vi "Get Time.vi"(9 "Next State in":T1, 10 "Current State":T1, 11 "State Start Time in":u32) -> (1 "Next State out":T1, 2 "Reset":bool, 3 "State Start Time out":u32)   [LabVIEW 2013]
uses:
  Auto Two Ball States.ctl
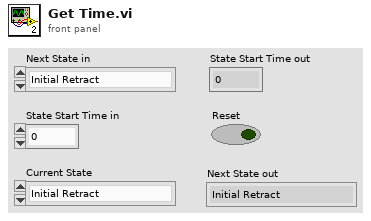
[diagram p1: front panel]
types:
  T1 = typedef "Auto Two Ball States.ctl" = enum16{"Initial Retract", "Initial Retract Wait", "First Shot: Wait for ball", "First Shot: Shoot", "Second Shot: Wait for Arm", "Grab Second Ball", "Grab Second Ball Wait", "Second Shot: Wait for ball", "Second Shot: Shoot", "Drive Forward", "Finish"}
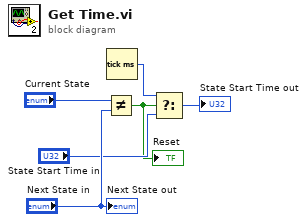
[diagram p0: block diagram]
diagram:
  n1 = Not Equal?(x="Current State", y="Next State in") -> (x != y?=w3:bool)
  "Reset" <- w3
  n2 = Tick Count (ms)() -> (millisecond timer value=w1:u32)
  n3 = Select(t=w1, s=w3, f="State Start Time in") -> (s? t:f=→"State Start Time out":u32)
  "Next State out" <- "Next State in"
